vi "video.create_set_property.vi"(8 "error in":errorcluster, 11 "VideoCreateStaging in":refnum<class "VideoCreateStaging.lvclass">) -> (0 "error out":errorcluster, 3 "VideoCreateStaging out":refnum<class "VideoCreateStaging.lvclass">)   [LabVIEW 2020, in "VideoCreateStaging.lvclass"]
doc: "Sets a property (key/value pair) on the video being created."
uses:
  VideoCreateStaging.lvclass
  VideoCreateStaging.lvclass/VideoCreateStaging.ctl
  client.lvlib
panel:
  in  "key":string
  in  "value":string
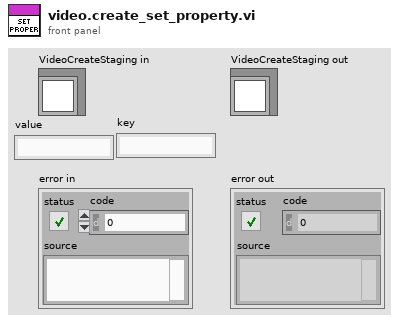
[diagram p1: front panel]
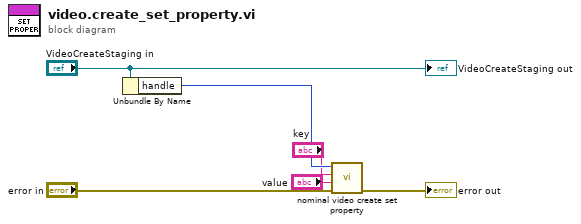
[diagram p0: block diagram]
diagram:
  n1 = Unbundle By Name("VideoCreateStaging in") -> ("handle"=w4:i32)
  n2 = call "nominal video create set property.vi"("error in (no error)"="error in", "value"="value", "key"="key", "staging"=w4) -> ("error out"=→"error out":errorcluster)  [unwired: 6 in, 1 out]
  "VideoCreateStaging out" <- "VideoCreateStaging in"
